vi "EF_CalcMinDelay.vi"(7 "MinDelays":dbl[](array[numeric]), 9 "Scale.Minimum in":dbl, 11 "Scale.Maximum in":dbl) -> (1 "Scale.Minimum out":dbl, 2 "rescale":bool, 3 "Scale.Maximum out":dbl)   [LabVIEW 2017]
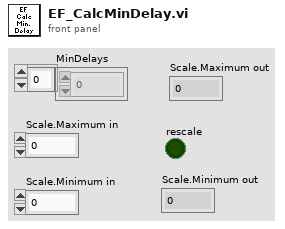
[diagram p1: front panel]
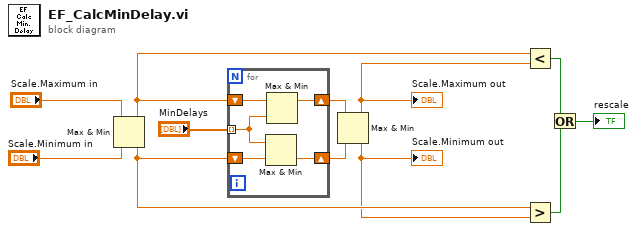
[diagram p0: block diagram]
diagram:
  n1 = Max & Min(x="Scale.Maximum in", y="Scale.Minimum in") -> (max(x,y)=w7:dbl, min(x,y)=w5:dbl)
  n2 = for {
    tunnel: "MinDelays" -> [w15] mode=indexing
    shift-right: [w17] -> w10
    shift-left: w7 -> [w16]
    shift-right: [w14] -> w11
    shift-left: w5 -> [w13]
    n3 = Max & Min(x=w15, y=w13) -> (min(x,y)=w14:dbl)  [unwired: 1 out]
    n4 = Max & Min(x=w16, y=w15) -> (max(x,y)=w17:dbl)  [unwired: 1 out]
  }
  n5 = Max & Min(x=w10, y=w11) -> (max(x,y)=w6:dbl, min(x,y)=w4:dbl)
  "Scale.Minimum out" <- w4
  "Scale.Maximum out" <- w6
  n6 = Less?(x=w7, y=w6) -> (x < y?=w3:bool)
  n7 = Greater?(x=w5, y=w4) -> (0:w2:bool)
  n8 = Or(x=w3, y=w2) -> (x .or. y?=→"rescale":bool)
